vi "GetType.vi"(8 "error in (no error)":errorcluster, 11 "Configure Sample Rate [ARB] Msg in":refnum<class "Configure Sample Rate [ARB] Msg.lvclass">) -> (0 "error out":errorcluster, 2 "Data Sample":variant, 3 "Configure Sample Rate [ARB] Msg out":refnum<class "Configure Sample Rate [ARB] Msg.lvclass">)   [LabVIEW 2014, in "CS++Fgen.lvlib" / "Configure Sample Rate [ARB] Msg.lvclass"]
doc: "This VI delivers a sample of the data type format the message expects."
uses:
  Configure Sample Rate [ARB] Msg.lvclass
  Configure Sample Rate [ARB] Msg.lvclass/Configure Sample Rate [ARB] Msg.ctl
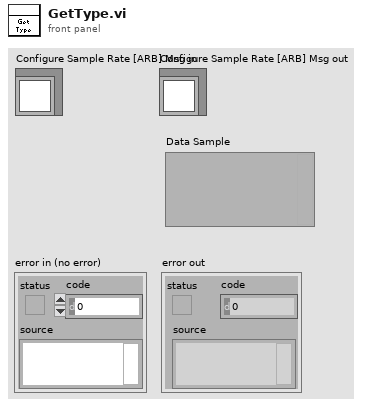
[diagram p1: front panel]
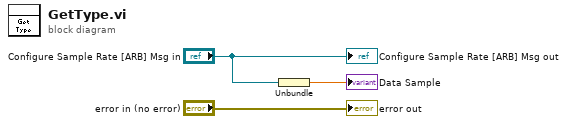
[diagram p0: block diagram]
diagram:
  n1 = Unbundle("Configure Sample Rate [ARB] Msg in") -> (→"Data Sample":dbl[unit])
  "error out" <- "error in (no error)"
  "Configure Sample Rate [ARB] Msg out" <- "Configure Sample Rate [ARB] Msg in"
